vi "Build Generic I2C Linux.vi"(7 "Read":bool, 8 "Bus Number":u8=2, 9 "Payload":u8[](array[numeric])=[10, 11, 10, 13, 11, 10, 11, 14] format="%.0x", 10 "7 bit Address":u8=64 format="%.0x", 11 "pcap Parse and Build in":refnum<class "pcap_Parse_Build_CIF.lvclass">) -> (2 "I2C Packet":u8[](array[numeric])=[231, 76, 198, 103, 241, 40, 73, 51, 14, 0, 0, 0, 14, 0, 0, 0, 2, 0, 0, 0, 0, 128, 10, 11, 10, 13, 11, 10, 11, 14] format="%.0x", 3 "pcap Parse and Build out":refnum<class "pcap_Parse_Build_CIF.lvclass">)   [LabVIEW 2021, in "pcap_Parse_Build_CIF.lvclass"]
uses:
  pcap_Parse_Build_CIF.lvclass
  pcap_Parse_Build_CIF.lvclass/pcap_Parse_Build_CIF.ctl
  <vilib>/CIF Foundation/CIF Utilities/Time/Time_CIF_U.lvlib
  Typedef/I2C Linux Header.ctl
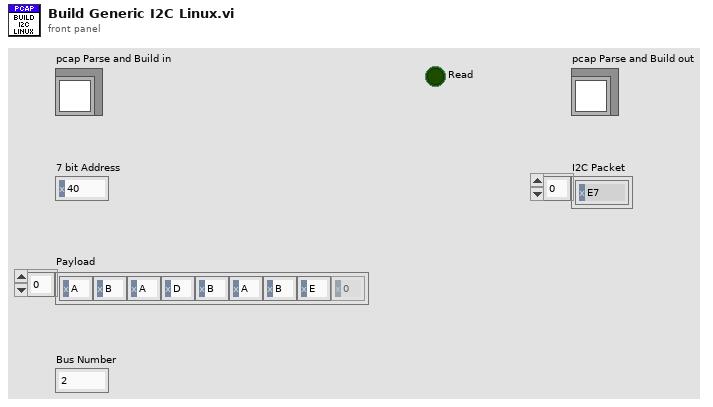
[diagram p1: front panel]
types:
  T1 = typedef "pcap_Parse_Build_CIF.lvclass/I2C Linux Header.ctl" = cluster{"Bus Number and Event Flag":u8, "Flags":u32, "HW Address":u8}
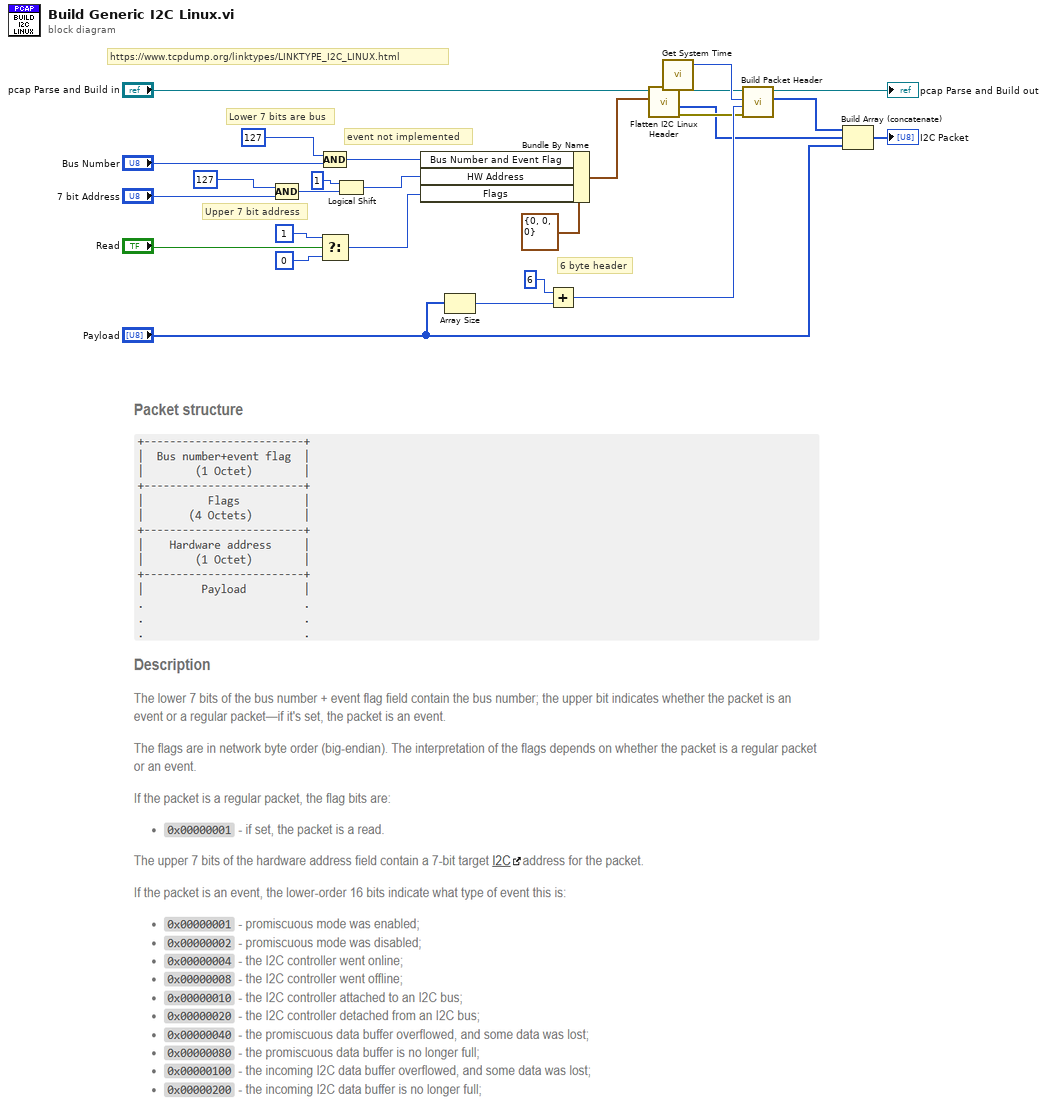
[diagram p0: block diagram]
diagram:
  # "event not implemented"
  # "Upper 7 bit address"
  # "https://www.tcpdump.org/linktypes/LINKTYPE_I2C_LINUX.html"
  # "6 byte header"
  # "Lower 7 bits are bus"
  n1 = Compound Arithmetic op=AND(u8 127, "7 bit Address") -> (w4:u8)
  n2 = Select(t=u32 1, s="Read", f=u32 0) -> (s? t:f=w5:u32)
  n3 = Compound Arithmetic op=AND(u8 127, "Bus Number") -> (w10:u8)
  n4 = Logical Shift(y=i16 1, x=w4) -> (x << y=w3:u8)
  n5 = Bundle By Name(cluster=T1 {"Bus Number and Event Flag"=0, "Flags"=0, "HW Address"=0} ("I2C Linux Header in 2"), "Bus Number and Event Flag"=w10, "HW Address"=w3, "Flags"=w5) -> (w15:T1)
  n6 = Array Size(array="Payload") -> (size(s)=w14:i32)
  n7 = Add(x=6, y=w14) -> (x+y=w24:i32)
  n8 = call "Flatten I2C Linux Header.vi"("I2C Linux Header in"=w15, "pcap Parse and Build in"="pcap Parse and Build in") -> ("error out"=w17:errorcluster, "Flattened Data out"=w16:u8[], "pcap Parse and Build out"=w18:refnum<class "pcap_Parse_Build_CIF.lvclass">)  [unwired: 6 in, 1 out]
  n9 = call <vilib>:"Get System Time.vi"() -> ("Time (ns)"=w23:i64)  [unwired: 5 in]
  n10 = call "Build Packet Header.vi"("error in (no error)"=w17, "Length"=w24, "TAI Time (ns)"=w23, "pcap Parse and Build in"=w18) -> ("Flattened Data out"=w22:u8[], "pcap Parse and Build out"=→"pcap Parse and Build out":refnum<class "pcap_Parse_Build_CIF.lvclass">)  [unwired: 5 in, 1 out]
  n11 = Build Array (concatenate)(w22, w16, "Payload") -> (→"I2C Packet":u8[])
